vi "Query Form SQL.vi"(2 "SQL query":string, 3 "SQL ID":string) -> (0 "error out":errorcluster, 1 "data":string[][](table))   [LabVIEW 2018]
uses:
  <vilib>/addons/database/Connection.llb/DB Tools Open Connec (String).vi
  <vilib>/addons/database/Connection.llb/Conn Execute.vi
  <vilib>/addons/database/Recordset.llb/Rec Fetch Recordset Data (R).vi
  <vilib>/addons/database/Recordset.llb/Rec Destroy - Connection.vi
  <vilib>/addons/database/_DB Variant To Data/Database Variant To Data.xnode
  <vilib>/addons/database/NI_Database_API.lvlib
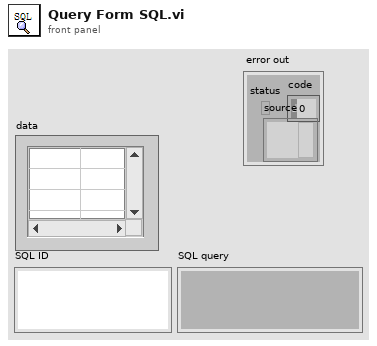
[diagram p1: front panel]
types:
  T1 = typedef "NI_Database_API.lvlib/Conn ObjectReference.ctl" = refnum<k1>
  T2 = typedef "NI_Database_API.lvlib/Rec ObjectReference.ctl" = refnum<k1>
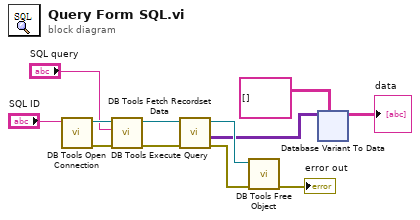
[diagram p0: block diagram]
diagram:
  n1 = call-poly <vilib>:"DB Tools Open Connection.vi"("connection information"="SQL ID") -> ("error out"=w10:errorcluster, "connection reference"=w12:T1)  [unwired: 7 in]
  n2 = call-poly <vilib>:"DB Tools Execute Query.vi"("error in (no error)"=w10, "SQL query"="SQL query", "connection reference"=w12) -> ("error out"=w9:errorcluster, "recordset reference"=w11:T2)  [unwired: 5 in]
  n3 = call-poly <vilib>:"DB Tools Fetch Recordset Data.vi"("error in (no error)"=w9, "recordset reference"=w11) -> ("error out"=w4:errorcluster, "recordset data"=w3:variant[][], "recordset reference out"=w8:T2)  [unwired: 3 in]
  n4 = call-poly <vilib>:"DB Tools Free Object.vi"("error in (no error)"=w4, "recordset reference"=w8) -> ("error out"=→"error out":errorcluster)  [unwired: 8 in, 1 out]
  n5 = xnode "Database Variant To Data"("database variant"=w3, "type"=string[][] []) -> ("data"=→"data":string[][])  [unwired: 1 in, 1 out]
